vi "Get UI References.vi"(8 "error in (no error)":errorcluster, 11 "VI reference":refnum<vi>) -> (0 "error out":errorcluster, 2 "reference out":refnum<vi>, 3 "Controls[]":refnum<vi>[](array[refnum]))   [LabVIEW 2020, in "UI Controls Manager.lvlib" / "uiControlsMgr.lvclass"]
uses:
  uiControlsMgr.lvclass
panel:
  out "Array":errorcluster[](array[cluster])
  out "Table":string[][](table)
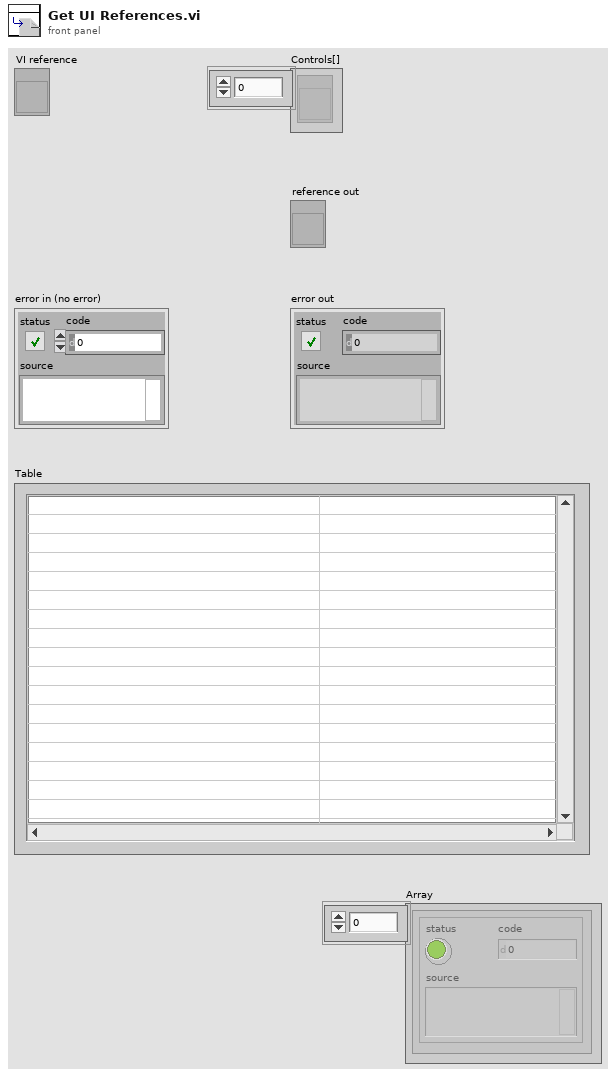
[diagram p1: front panel]
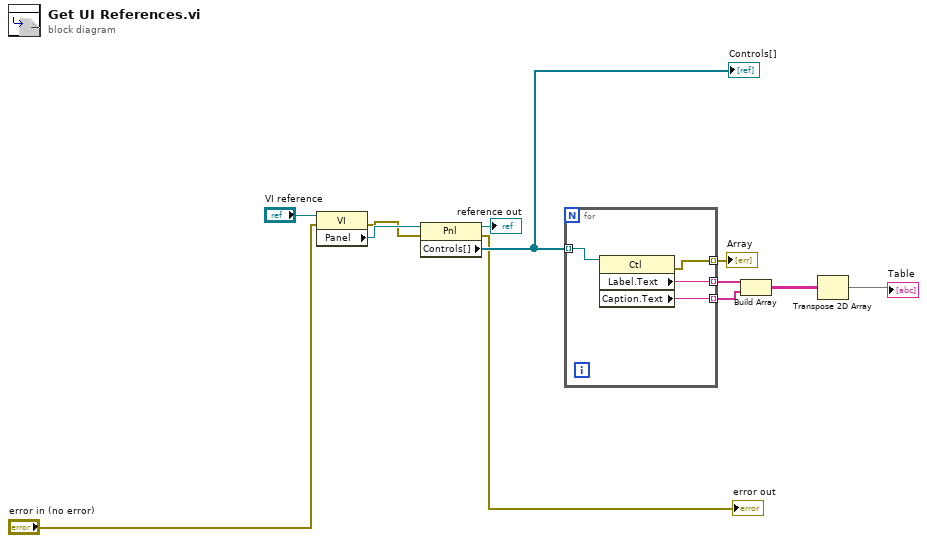
[diagram p0: block diagram]
diagram:
  n1 = property class="VI"(reference="VI reference", error in="error in (no error)") -> (error out=w5:errorcluster, "Panel"=w11:refnum<vi>)  [unwired: 1 out]
  n2 = property class="Pnl"(reference=w11, error in=w5) -> (reference out=→"reference out":refnum<vi>, error out=→"error out":errorcluster, "Controls[]"=w12:refnum<vi>[])
  "Controls[]" <- w12
  n3 = for {
    tunnel: w12 -> [w14] mode=indexing
    tunnel: [w16] -> w10 mode=indexing
    tunnel: [w15] -> w9 mode=indexing
    tunnel: [w13] -> w2 mode=indexing
    n4 = property class="Ctl"(reference=w14) -> (error out=w13:errorcluster, "Label.Text"=w16:string, "Caption.Text"=w15:string)  [unwired: 1 in, 1 out]
  }
  "Array" <- w2
  n5 = Build Array(w10, w9) -> (w8:string[][])
  n6 = Transpose 2D Array(2D array=w8) -> (transposed array=→"Table":string[][])
